vi "ErrorDefinitionSQLite_TestClass.vi"() -> ()   [LabVIEW 2018]
uses:
  ErrorContent.ctl
  ErrorDefinitionSQLite.lvclass
panel:
  out "Errors":T1
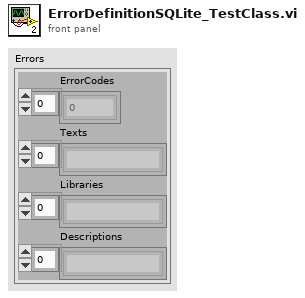
[diagram p1: front panel]
types:
  T1 = typedef "ErrorDefinitionSQLite.lvclass/ErrorContent.ctl" = cluster{"ErrorCodes":i32[], "Texts":string[], "Libraries":string[], "Descriptions":string[]}
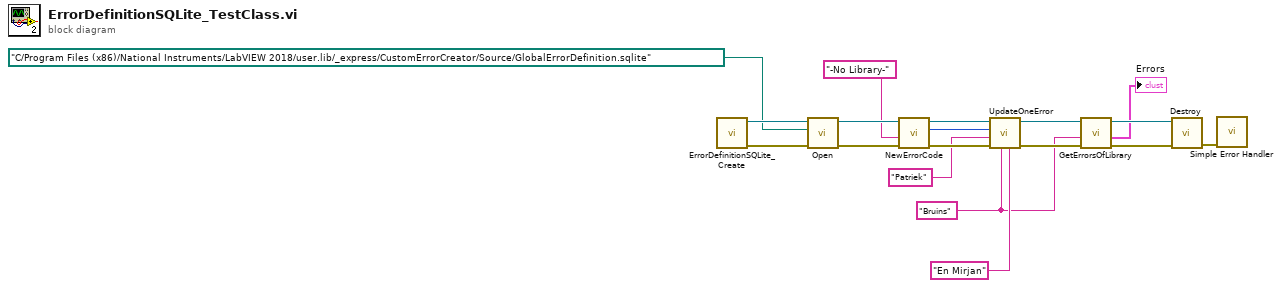
[diagram p0: block diagram]
diagram:
  w4 = "Bruins" ("Library")
  n1 = call "ErrorDefinitionSQLite_Create.vi"() -> ("ErrorOut"=w17:errorcluster, "Reference out"=w18:refnum<class "ErrorDefinitionSQLite.lvclass">)  [unwired: 10 in]
  n2 = call-dynamic "Open.vi"("ErrorIn"=w17, "Path"=path "C:/Program Files (x86)/National Instruments/LabVIEW 2018/user.lib/_express/CustomErrorCreator/Source/GlobalErrorDefinition.sqlite", "ReferenceIn"=w18) -> ("ErrorOut"=w15:errorcluster, "ReferenceOut"=w16:refnum<class "ErrorDefinitionSQLite.lvclass">)  [unwired: 7 in]
  n3 = call-dynamic "NewErrorCode.vi"("ErrorIn"=w15, "LibraryName"="-No Library-", "ReferenceIn"=w16) -> ("ErrorOut"=w13:errorcluster, "NewErrorCode"=w7:i32, "ReferenceOut"=w14:refnum<class "ErrorDefinitionSQLite.lvclass">)  [unwired: 6 in]
  n4 = call-dynamic "UpdateOneError.vi"("Description"="En Mirjan", "Library"=w4, "ErrorIn"=w13, "Text"="Patriek", "ErrorCode"=w7, "ReferenceIn"=w14) -> ("ErrorOut"=w11:errorcluster, "ReferenceOut"=w12:refnum<class "ErrorDefinitionSQLite.lvclass">)  [unwired: 4 in]
  n5 = call-dynamic "GetErrorsOfLibrary.vi"("ErrorIn"=w11, "LibraryName"=w4, "ReferenceIn"=w12) -> ("ErrorOut"=w9:errorcluster, "Errors"=→"Errors":T1, "ReferenceOut"=w10:refnum<class "ErrorDefinitionSQLite.lvclass">)  [unwired: 6 in]
  n6 = call-dynamic "Destroy.vi"("ErrorIn"=w9, "Reference in"=w10) -> ("ErrorOut"=w2:errorcluster)  [unwired: 8 in, 1 out]
  n7 = call <vilib>:"Simple Error Handler.vi"("error in (no error)"=w2) -> ()  [unwired: 4 in, 5 out]
